vi "Get Configuration Metadata.vi"(8 "error in (no error)":errorcluster) -> (0 "error out":errorcluster, 3 "Metadata Value":T1(array[cluster]))   [LabVIEW 2020, in "CancellableMeasurementProxy.lvlib"]
uses:
  CancellableMeasurementProxy.lvlib
  Configuration Metadata.ctl
  TypeDefs/Type Specialization.ctl
  TypeDefs/Key.ctl
  c705a3e4-b692-4185-b671-4f4934be27f2.vi
  <vilib>/Utility/Data Type/Get Type Definition Path.vi
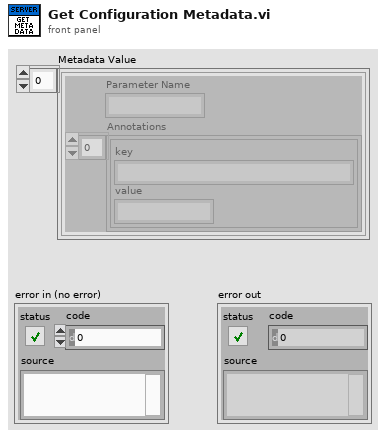
[diagram p1: front panel]
types:
  T1 = cluster{"Parameter Name":string, "Annotations":cluster{"key":string, "value":string}[]}[]
  T2 = typedef "CancellableMeasurementProxy.lvlib/Configuration Metadata.ctl" = cluster{"Parameter Name":string, "Type Specialization":T3, "Annotations":cluster{"Key":T4, "Value":string}[]}[]
  T3 = typedef "CancellableMeasurementProxy.lvlib/Type Specialization.ctl" = enum16{"none", "pin"}
  T4 = typedef "CancellableMeasurementProxy.lvlib/Key.ctl" = enum16{"none", "pin.instrument_type"}
  T5 = cluster{"Parameter Name":string, "Annotations":cluster{"Value":string, "Value 2":string}[]}
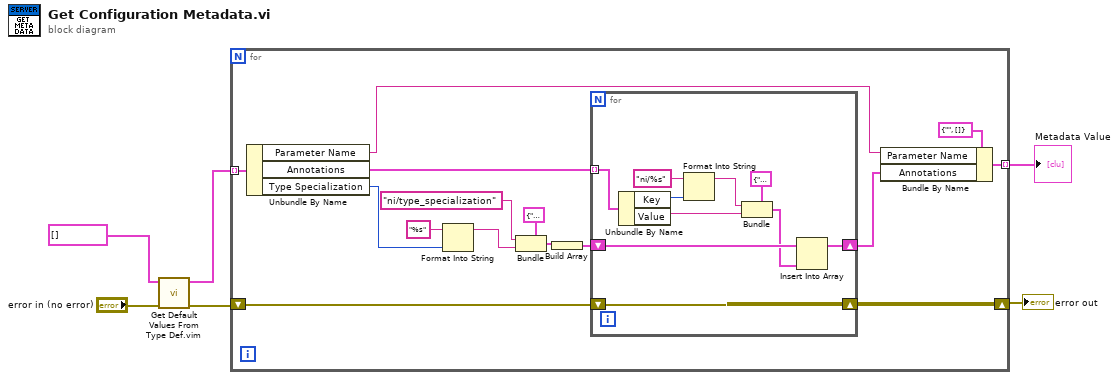
[diagram p0: block diagram]
diagram:
  n1 = call "Get Default Values From Type Def.vim"("error in (no error)"="error in (no error)", "Type Def"=T2 [] ("Configuration Metadata")) -> ("error out"=w1:errorcluster, "Default Values"=w2:T2)  [unwired: 8 in]
  n2 = for {
    tunnel: w2 -> [w21] mode=indexing
    shift-right: [w17] -> w4
    shift-left: w1 -> [w18]
    tunnel: [w19] -> w3 mode=indexing
    n3 = Unbundle By Name(w21) -> ("Parameter Name"=w7:string, "Annotations"=w11:cluster{"Key":T4, "Value":string}[], "Type Specialization"=w15:T3)
    n4 = Format Into String(format string="%s", w15) -> (resulting string=w13:string)  [unwired: 2 in, 1 out]
    n5 = Bundle(cluster=cluster{"Value":string, "Value 2":string} {"Value"="", "Value 2"=""} ("Cluster 2"), "Value"="ni/type_specialization", "Value 2"=w13) -> (w8:cluster{"Value":string, "Value 2":string})
    n6 = Build Array(w8) -> (w9:cluster{"Value":string, "Value 2":string}[])
    n7 = for {
      shift-right: [w31] -> w17
      shift-left: w18 -> [w31]
      tunnel: w11 -> [w30] mode=indexing
      shift-right: [w22] -> w10
      shift-left: w9 -> [w24]
      n8 = Unbundle By Name(w30) -> ("Key"=w28:T4, "Value"=w25:string)
      n9 = Format Into String(format string="ni/%s", w28) -> (resulting string=w26:string)  [unwired: 2 in, 1 out]
      n10 = Bundle(cluster=cluster{"Value":string, "Value 2":string} {"Value"="", "Value 2"=""} ("Cluster 2"), "Value"=w26, "Value 2"=w25) -> (w23:cluster{"Value":string, "Value 2":string})
      n11 = Insert Into Array(array=w24, new element=w23) -> (w22:cluster{"Value":string, "Value 2":string}[])  [unwired: 1 in]
    }
    n12 = Bundle By Name(cluster=T5 {"Parameter Name"="", "Annotations"=[]} ("Cluster"), "Parameter Name"=w7, "Annotations"=w10) -> (w19:T5)
  }
  "error out" <- w4
  "Metadata Value" <- w3
